vi "SaveNewPAQtags.vi"(8 "error in (no error)":errorcluster, 10 "TAGpropertyEdit":T1 {"TAGprop"."TagFunc" format="%08x"; "TAGprop"."RangeL" format="%.2f"; "TAGprop"."RangeH" format="%.2f"}, 11 "DBAL-BIN in":refnum<class "DBAL-BIN.lvclass">) -> (0 "error out":errorcluster, 3 "DBAL-BIN out":refnum<class "DBAL-BIN.lvclass">)   [LabVIEW 2020, in "Sgraph_lib_V1.lvlib" / "DBAL-BIN.lvclass"]
doc: "Save Binary TAG to PAQprops.ini file"
uses:
  DBAL-BIN.lvclass
  controls/DBAL_TAGpropEdit.ctl
  Common/controls/typedef_com_TagProp.ctl
  DBAL-BIN.lvclass/DBAL-BIN.ctl
  <vilib>/Utility/error.llb/Error Cluster From Error Code.vi
  <vilib>/ErrorRing/Error Ring.xnode
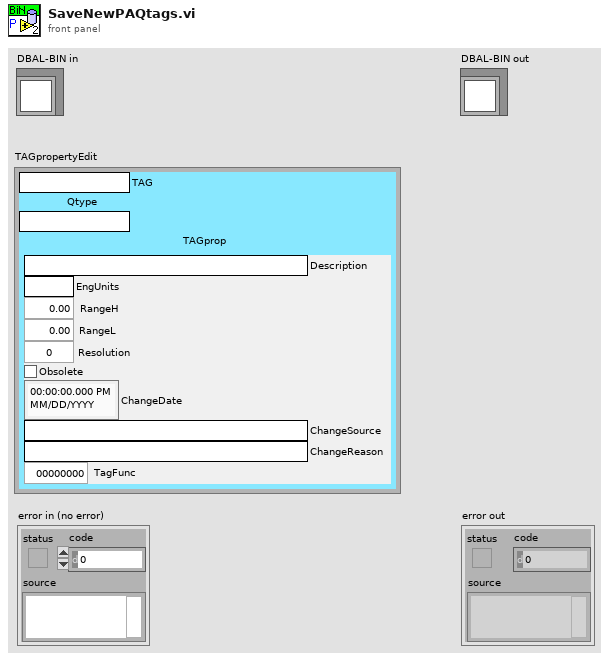
[diagram p1: front panel]
types:
  T1 = typedef "DBAL_TAGpropEdit.ctl" = cluster{"TAG":string, "Qtype":string, "TAGprop":T2}
  T2 = typedef "typedef_com_TagProp.ctl" = cluster{"Description":string, "EngUnits":string, "RangeH":dbl, "RangeL":dbl, "Resolution":i32, "Obsolete":bool, "ChangeDate":timestamp, "ChangeSource":string, "ChangeReason":string, "TagFunc":u32}
  T3 = enum16{"open", "replace", "create", "open or create", "replace or create", "replace or create with confirmation"}
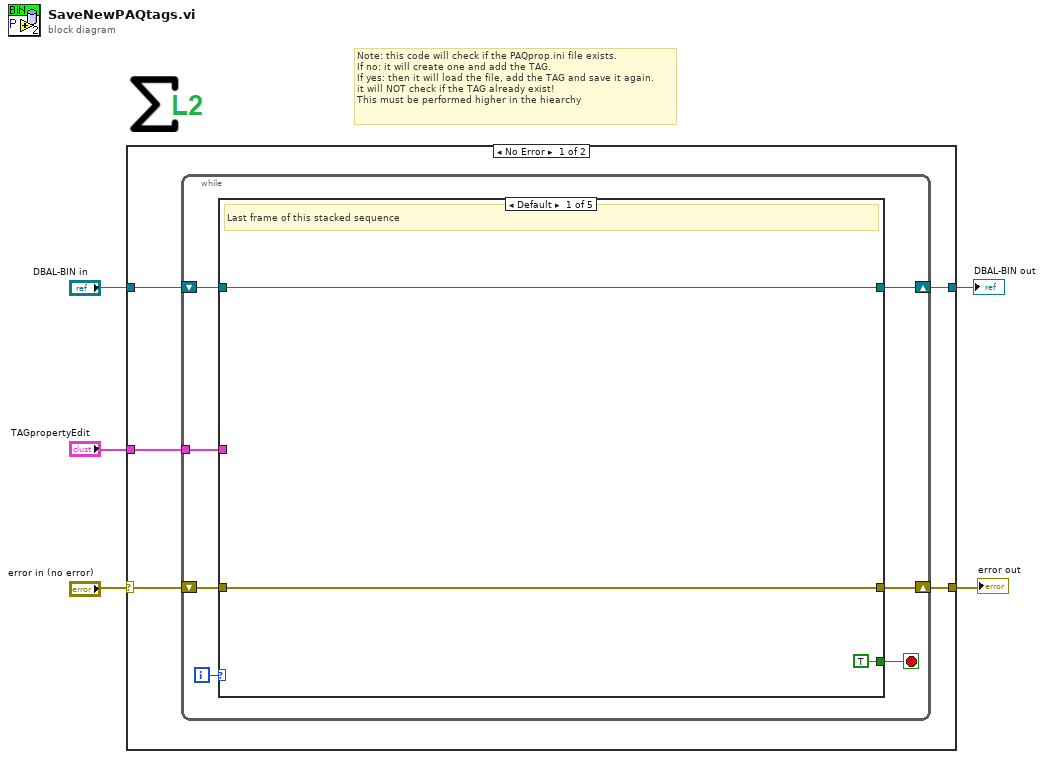
[diagram p0: block diagram]
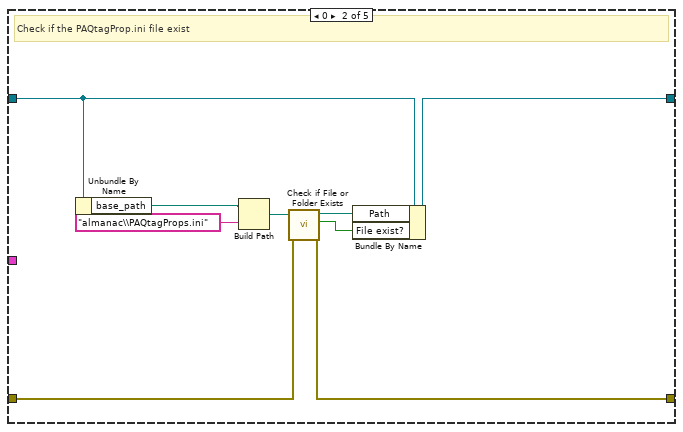
[diagram p2: hidden frame]
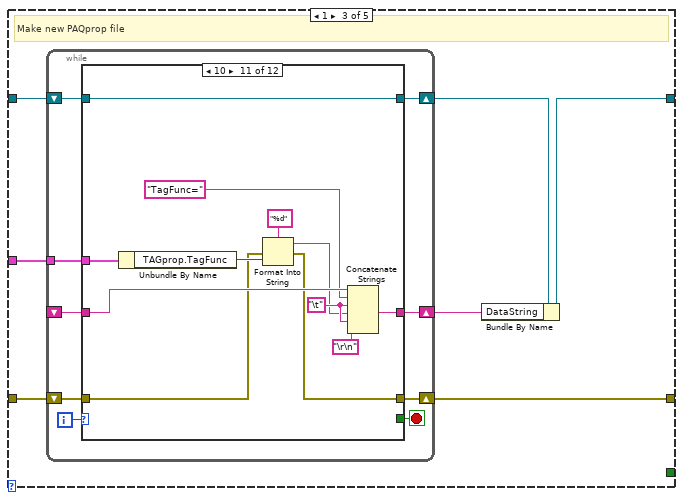
[diagram p3: hidden frame]
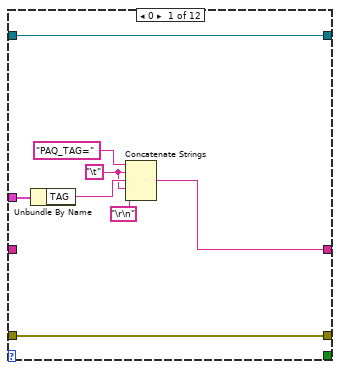
[diagram p4: hidden frame]
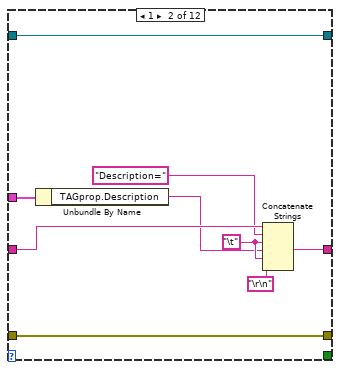
[diagram p5: hidden frame]
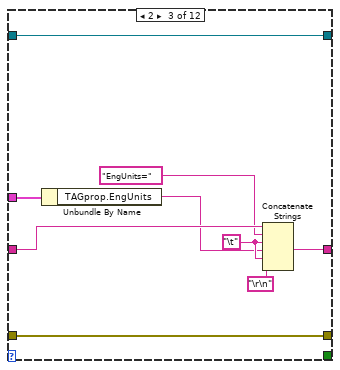
[diagram p6: hidden frame]
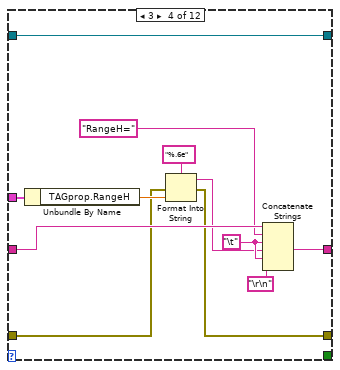
[diagram p7: hidden frame]
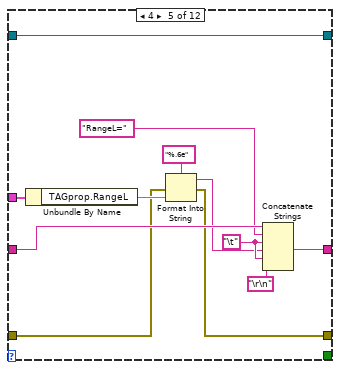
[diagram p8: hidden frame]
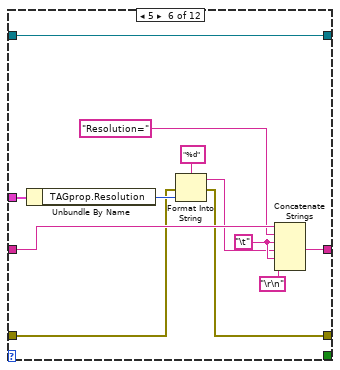
[diagram p9: hidden frame]
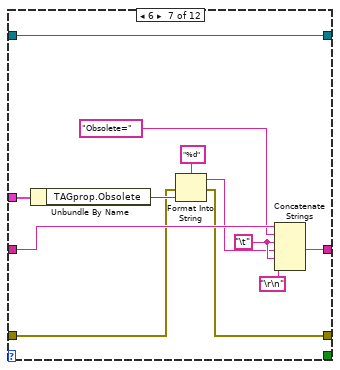
[diagram p10: hidden frame]
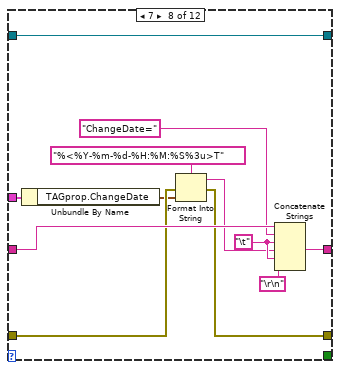
[diagram p11: hidden frame]
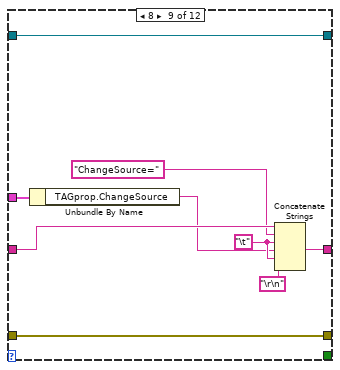
[diagram p12: hidden frame]
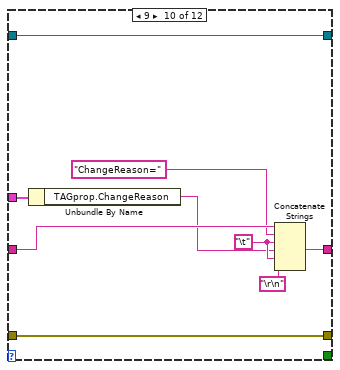
[diagram p13: hidden frame]
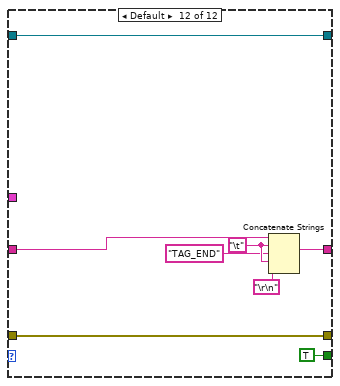
[diagram p14: hidden frame]
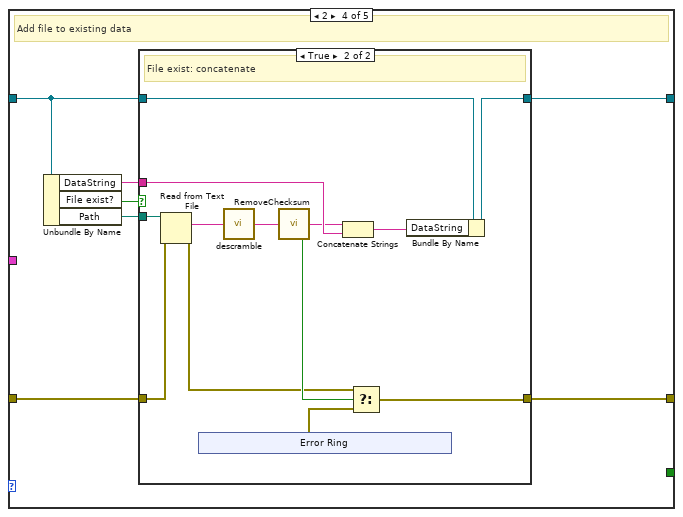
[diagram p15: hidden frame]
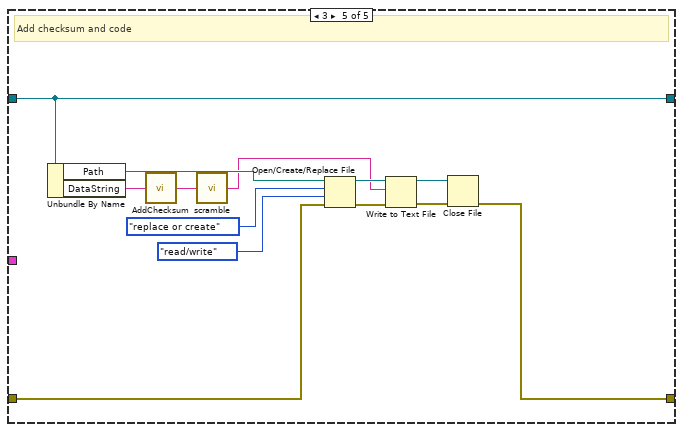
[diagram p17: hidden frame]
diagram:
  # "Note: this code will check if the PAQprop.ini file exists.\nIf no: it will create one and add the TAG.\nIf yes: then it will load the file, add the TAG and save it again.\nit will NOT check if the TAG already exist!\nThis must be performed higher in the hiearchy"
  n1 = case shown="No Error" "error in (no error)" {
    selector: "error in (no error)" -> [w9 w211]
    tunnel: [w7 w211] -> w2
    tunnel: [w8 w210] -> w3
    tunnel: "DBAL-BIN in" -> [w10 w210]
    tunnel: "TAGpropertyEdit" -> [w6 _]
    frame No Error {
      n2 = while {
        shift-right: [w13] -> w8
        shift-left: w10 -> [w15]
        shift-right: [w12] -> w7
        shift-left: w9 -> [w14]
        tunnel: w6 -> [w11]
        i -> [w17]
        stop <- w16 stop-if-true
        n3 = case shown="Default" w17 {
          tunnel: [TRUE _ _ _ _] -> w16
          tunnel: w15 -> [w18 w22 w35 w175 w209]
          tunnel: w14 -> [w19 w27 w36 w174 w203]
          tunnel: [w18 w23 w30 w173 w209] -> w13
          tunnel: [w19 w26 w33 w172 w197] -> w12
          tunnel: w11 -> [_ _ w34 _ _]
          frame Default {
            # "Last frame of this stacked sequence"
          }
          frame 0 {
            # "Check if the PAQtagProp.ini file exist"
            n4 = Unbundle By Name(w22) -> ("base_path"=w21:path)
            n5 = Build Path(base path=w21, name or relative path="almanac\\PAQtagProps.ini") -> (appended path=w28:path)
            n6 = call <vilib>:"Check if File or Folder Exists.vi"("error in (no error)"=w27, "path"=w28) -> ("error out"=w26:errorcluster, "file or folder exists?"=w24:bool, "dup path"=w25:path)  [unwired: 7 in]
            n7 = Bundle By Name(cluster=w22, "Path"=w25, "File exist?"=w24) -> (w23:refnum<class "DBAL-BIN.lvclass">)
          }
          frame 1 {
            # "Make new PAQprop file"
            n8 = while {
              shift-right: [w42] -> w31
              shift-left: w35 -> [w43]
              shift-right: [w41] -> w33
              shift-left: w36 -> [w44]
              tunnel: w34 -> [w40]
              shift-right: [w38] -> w32
              shift-left: _ -> [w39]
              i -> [w45]
              stop <- w37 stop-if-true
              n9 = case shown="10" w45 {
                tunnel: w44 -> [w52 w61 w70 w75 w87 w99 w111 w124 w133 w142 w152 w168]
                tunnel: w43 -> [w53 w62 w71 w83 w95 w107 w119 w131 w140 w149 w161 w169]
                tunnel: [w53 w62 w71 w83 w95 w107 w119 w131 w140 w149 w161 w169] -> w42
                tunnel: [w52 w61 w70 w74 w86 w98 w110 w123 w133 w142 w151 w168] -> w41
                tunnel: w40 -> [w51 w60 w69 w82 w94 w106 w118 w130 w139 w148 w160 _]
                tunnel: w39 -> [_ w57 w66 w79 w91 w103 w115 w127 w136 w145 w157 w163]
                tunnel: [w49 w54 w63 w77 w89 w101 w113 w125 w134 w143 w155 w162] -> w38
                tunnel: [_ _ _ _ _ _ _ _ _ _ _ TRUE] -> w37
                frame 0 {
                  w47 = "\t"
                  n10 = Unbundle By Name(w51) -> ("TAG"=w50:string)
                  n11 = Concatenate Strings("PAQ_TAG=", w47, w50, w47, "\r\n") -> (w49:string)
                }
                frame 1 {
                  w58 = "\t"
                  n12 = Unbundle By Name(w60) -> ("TAGprop.Description"=w55:string)
                  n13 = Concatenate Strings(w57, "Description=", w58, w55, w58, "\r\n") -> (w54:string)
                }
                frame 2 {
                  w67 = "\t"
                  n14 = Unbundle By Name(w69) -> ("TAGprop.EngUnits"=w64:string)
                  n15 = Concatenate Strings(w66, "EngUnits=", w67, w64, w67, "\r\n") -> (w63:string)
                }
                frame 3 {
                  w80 = "\t"
                  n16 = Unbundle By Name(w82) -> ("TAGprop.RangeH"=w76:dbl)
                  n17 = Format Into String(format string="%.6e", error in=w75, w76) -> (resulting string=w72:string, error out=w74:errorcluster)  [unwired: 1 in]
                  n18 = Concatenate Strings(w79, "RangeH=", w80, w72, w80, "\r\n") -> (w77:string)
                }
                frame 4 {
                  w92 = "\t"
                  n19 = Unbundle By Name(w94) -> ("TAGprop.RangeL"=w88:dbl)
                  n20 = Format Into String(format string="%.6e", error in=w87, w88) -> (resulting string=w84:string, error out=w86:errorcluster)  [unwired: 1 in]
                  n21 = Concatenate Strings(w91, "RangeL=", w92, w84, w92, "\r\n") -> (w89:string)
                }
                frame 5 {
                  w104 = "\t"
                  n22 = Unbundle By Name(w106) -> ("TAGprop.Resolution"=w100:i32)
                  n23 = Format Into String(format string="%d", error in=w99, w100) -> (resulting string=w96:string, error out=w98:errorcluster)  [unwired: 1 in]
                  n24 = Concatenate Strings(w103, "Resolution=", w104, w96, w104, "\r\n") -> (w101:string)
                }
                frame 6 {
                  w116 = "\t"
                  n25 = Unbundle By Name(w118) -> ("TAGprop.Obsolete"=w112:bool)
                  n26 = Format Into String(format string="%d", error in=w111, w112) -> (resulting string=w108:string, error out=w110:errorcluster)  [unwired: 1 in]
                  n27 = Concatenate Strings(w115, "Obsolete=", w116, w108, w116, "\r\n") -> (w113:string)
                }
                frame 7 {
                  w128 = "\t"
                  n28 = Unbundle By Name(w130) -> ("TAGprop.ChangeDate"=w120:timestamp)
                  n29 = Format Into String(format string="%<%Y-%m-%d-%H:%M:%S%3u>T", error in=w124, w120) -> (resulting string=w121:string, error out=w123:errorcluster)  [unwired: 1 in]
                  n30 = Concatenate Strings(w127, "ChangeDate=", w128, w121, w128, "\r\n") -> (w125:string)
                }
                frame 8 {
                  w137 = "\t"
                  n31 = Unbundle By Name(w139) -> ("TAGprop.ChangeSource"=w132:string)
                  n32 = Concatenate Strings(w136, "ChangeSource=", w137, w132, w137, "\r\n") -> (w134:string)
                }
                frame 9 {
                  w146 = "\t"
                  n33 = Unbundle By Name(w148) -> ("TAGprop.ChangeReason"=w141:string)
                  n34 = Concatenate Strings(w145, "ChangeReason=", w146, w141, w146, "\r\n") -> (w143:string)
                }
                frame 10 {
                  w158 = "\t"
                  n35 = Unbundle By Name(w160) -> ("TAGprop.TagFunc"=w153:u32)
                  n36 = Format Into String(format string="%d", error in=w152, w153) -> (resulting string=w150:string, error out=w151:errorcluster)  [unwired: 1 in]
                  n37 = Concatenate Strings(w157, "TagFunc=", w158, w150, w158, "\r\n") -> (w155:string)
                }
                frame Default {
                  w166 = "\t"
                  n38 = Concatenate Strings(w163, w166, "TAG_END", w166, "\r\n") -> (w162:string)
                }
              }
            }
            n39 = Bundle By Name(cluster=w31, "DataString"=w32) -> (w30:refnum<class "DBAL-BIN.lvclass">)
          }
          frame 2 {
            # "Add file to existing data"
            n40 = Unbundle By Name(w175) -> ("DataString"=w171:string, "File exist?"=w176:bool, "Path"=w170:path)
            n41 = case shown="True" w176 {
              tunnel: w175 -> [w178 w187]
              tunnel: w174 -> [w177 w190]
              tunnel: [w178 w186] -> w173
              tunnel: [w177 w181] -> w172
              tunnel: w171 -> [_ w189]
              tunnel: w170 -> [_ w191]
              frame False {
                # "File does not exist : nothing to add"
              }
              frame True {
                # "File exist: concatenate"
                n42 = Read from Text File(file (use dialog)=w191, error in=w190) -> (text=w185:string, error out=w180:errorcluster)  [unwired: 2 in, 2 out]
                n43 = xnode "Error Ring"() -> ("error out"=w179:errorcluster)
                n44 = call "descramble.vi"("scrambled"=w185) -> ("OUT"=w184:string)  [unwired: 6 in]
                n45 = call "RemoveChecksum.vi"("IN"=w184) -> ("Check OK?"=w182:bool, "OUT"=w183:string)  [unwired: 3 in]
                n46 = Concatenate Strings(w183, w189) -> (w188:string)
                n47 = Select(t=w180, s=w182, f=w179) -> (s? t:f=w181:errorcluster)
                n48 = Bundle By Name(cluster=w187, "DataString"=w188) -> (w186:refnum<class "DBAL-BIN.lvclass">)
              }
            }
          }
          frame 3 {
            # "Add checksum and code"
            n49 = Unbundle By Name(w209) -> ("Path"=w206:path, "DataString"=w208:string)
            n50 = call "AddChecksum.vi"("String IN"=w208) -> ("OUT"=w207:string)  [unwired: 8 in]
            n51 = call "scramble.vi"("clean"=w207) -> ("scrambled"=w200:string)  [unwired: 6 in]
            n52 = Open/Create/Replace File(file path (use dialog)=w206, error in=w203, operation (0:open)=T3."replace or create", access (0:read/write)=enum16{"read/write", "read-only", "write-only"}."read/write") -> (refnum out=w202:refnum<file>, error out=w201:errorcluster)  [unwired: 2 in, 1 out]
            n53 = Write to Text File(file (use dialog)=w202, text=w200, error in=w201) -> (refnum out=w198:refnum<file>, error out=w199:errorcluster)  [unwired: 1 in, 1 out]
            n54 = Close File(refnum=w198, error in=w199) -> (error out=w197:errorcluster)  [unwired: 1 out]
          }
        }
      }
    }
    frame Error {
    }
  }
  "error out" <- w2
  "DBAL-BIN out" <- w3
